vi "GetSetControlledStopParms.vi"(8 "error in":errorcluster, 9 "Input parms":T1 {"Controlled stop control mode (1=on; 0=off)" max=1 step=1; "Controlled stop deviation (0 - 999.9 deg C)" min=0 max=50 step=1 format="%0.1f"; "Controlled stop purge time (0-3600 seconds)" max=3600 step=1; "Controlled stop set point (0 - 50 deg C)" max=50 step=1; "Controlled stop mode (1=enable; 0=disable)" max=1 step=1}, 10 "get/set":T2, 11 "VISA resource name":refnum<visa-resource-name>) -> (0 "error out":errorcluster, 2 "Controlled stop parms response":string, 3 "VISA resource name out":refnum<visa-resource-name>)   [LabVIEW 2023, in "Thermotron 8800.lvlib"]
doc: "SSTP\nCAUTION: This command is included for advanced users.\nCommand name: Send or load controlled stop (safety stop) parameter values\nCommand type: Variable\nDescription: The query command causes the 8800 to return the values of the controlled stop parameters. The operation command sends new controlled stop parameter values. NOTE: Earlier software versions used the term safety stop instead of controlled stop.\nQuery syntax: SSTP?\nOperation syntax: SSTPm, sp, prg, dev, ctl\nWhere:\nm Controlled stop mode enabled (1) or disabled (0)\nsp Controlled stop set point (0-50 degrees C)\nprg Controlled stop purge time (0-3,600 seconds)\ndev Controlled stop deviation (0-999.9 degrees C)\nctl Controlled stop control mode on (1) or off (0)\nQuery example: SSTP?\n8800 response: 1,25.0,30, 2.5, 1 (Controlled stop mode is enabled, the controlled stop set point is 25°C, the controlled stop purge time is 30 seconds, the controlled stop deviation is 2.5°C, and controlled stop control mode is on.)\nOperation examples: SSTP1,30,10,5,1 (Enable controlled stop mode, set the controlled stop set point to 30°C, set the controlled stop purge time to 10 seconds, set the controlled stop deviation to 5°C, and turn on controlled stop control mode.)\nSSTP1 (Enable controlled stop mode. Leave the other parameters as they were.)\nSSTP0 (Disable controlled stop mode. Leave the other parameters as they were.)"
uses:
  Thermotron 8800.lvlib
  Private/get set.ctl
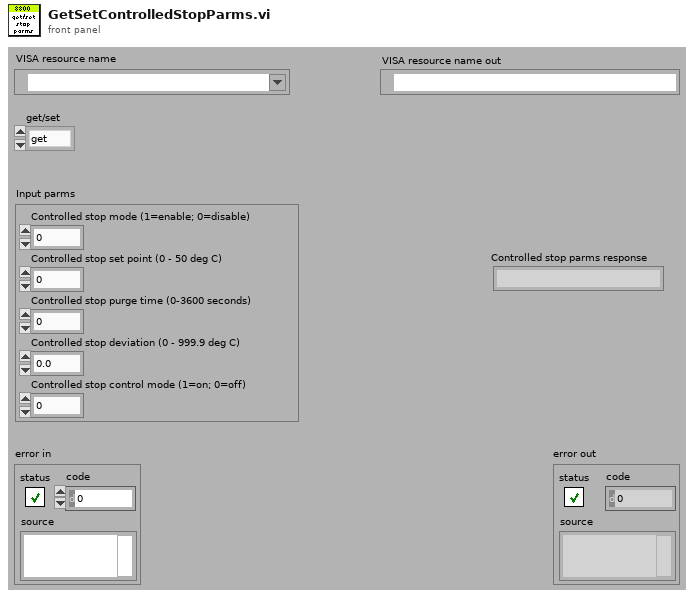
[diagram p1: front panel]
types:
  T1 = cluster{"Controlled stop mode (1=enable; 0=disable)":u8, "Controlled stop set point (0 - 50 deg C)":u8, "Controlled stop purge time (0-3600 seconds)":u16, "Controlled stop deviation (0 - 999.9 deg C)":sgl, "Controlled stop control mode (1=on; 0=off)":u8}
  T2 = typedef "Thermotron 8800.lvlib/get set.ctl" = enum16{"get", "set"}
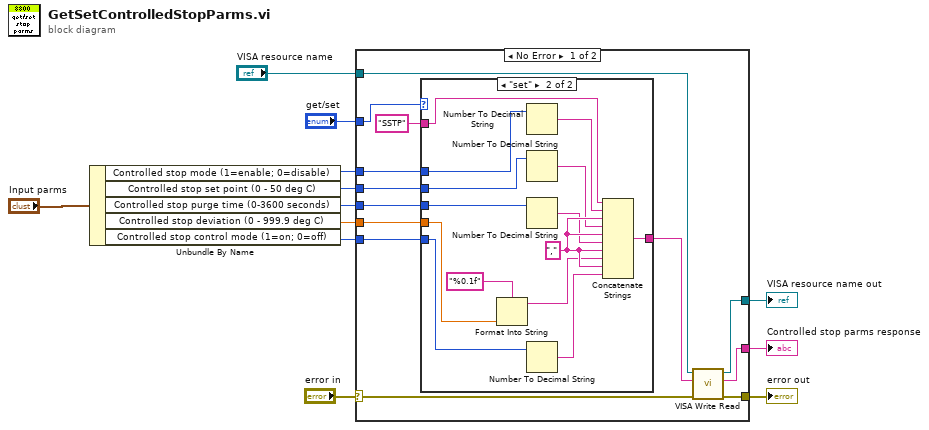
[diagram p0: block diagram]
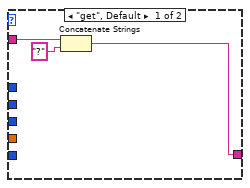
[diagram p2: hidden frame]
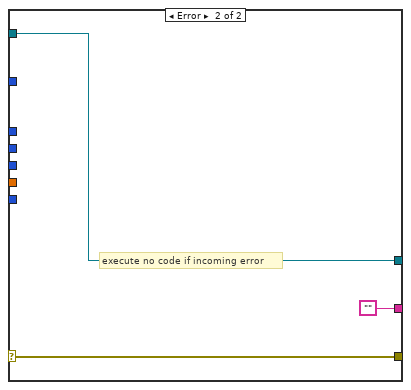
[diagram p3: hidden frame]
diagram:
  n1 = Unbundle By Name("Input parms") -> ("Controlled stop mode (1=enable; 0=disable)"=w5:u8, "Controlled stop set point (0 - 50 deg C)"=w4:u8, "Controlled stop purge time (0-3600 seconds)"=w3:u16, "Controlled stop deviation (0 - 999.9 deg C)"=w2:sgl, "Controlled stop control mode (1=on; 0=off)"=w1:u8)
  n2 = case shown="No Error" "error in" {
    selector: "error in" -> [w17 w44]
    tunnel: "get/set" -> [w25 _]
    tunnel: [w22 ""] -> w7
    tunnel: [w21 w44] -> w10
    tunnel: [w20 w45] -> w9
    tunnel: "VISA resource name" -> [w19 w45]
    tunnel: w5 -> [w18 _]
    tunnel: w4 -> [w16 _]
    tunnel: w3 -> [w15 _]
    tunnel: w2 -> [w14 _]
    tunnel: w1 -> [w13 _]
    frame No Error {
      n3 = case shown="\"set\"" w25 {
        tunnel: "SSTP" ("8800 Command") -> [w27 w42]
        tunnel: [w28 w41] -> w23
        tunnel: w18 -> [_ w39]
        tunnel: w16 -> [_ w30]
        tunnel: w15 -> [_ w36]
        tunnel: w14 -> [_ w34]
        tunnel: w13 -> [_ w32]
        frame "get", Default {
          n4 = Concatenate Strings(w27, "?" ("8800 Command")) -> (w28:string)
        }
        frame "set" {
          w38 = ","
          n5 = Format Into String(format string="%0.1f", w34) -> (resulting string=w33:string)  [unwired: 2 in, 1 out]
          n6 = Number To Decimal String(number=w39) -> (decimal integer string=w40:string)  [unwired: 1 in]
          n7 = Number To Decimal String(number=w30) -> (decimal integer string=w29:string)  [unwired: 1 in]
          n8 = Number To Decimal String(number=w36) -> (decimal integer string=w35:string)  [unwired: 1 in]
          n9 = Number To Decimal String(number=w32) -> (decimal integer string=w31:string)  [unwired: 1 in]
          n10 = Concatenate Strings(w42, w40, w38, w29, w38, w35, w38, w33, w38, w31) -> (w41:string)
        }
      }
      n11 = call "VISA Write Read.vi"("error in (no error)"=w17, "8800 Command"=w23, "VISA Refnum in"=w19) -> ("error out"=w21:errorcluster, "read buffer"=w22:string, "VISA Refnum out"=w20:refnum<visa-resource-name>)  [unwired: 6 in]
    }
    frame Error {
      # "execute no code if incoming error"
    }
  }
  "VISA resource name out" <- w9
  "error out" <- w10
  "Controlled stop parms response" <- w7
